vi "Untitled 1.vi"() -> ()   [LabVIEW 2021]
uses:
  <vilib>/numeric/Random Number (Range) U64.vi
  <vilib>/numeric/sub_Random U32.vi
panel:
  out "Tank":dbl(slide) scale=0.0..10.0
  in  "stop 2":bool
  out "Boolean":bool
  out "Knob":dbl(knob) scale=0.0..10.0
  out "Numeric":i32
  in  "stop":bool
  out "number":u64
  out "x+1":i32
  # "For loop"
  # "While loop"
  # "Example: Flat and stacked structures"
  # "Exercise 6"
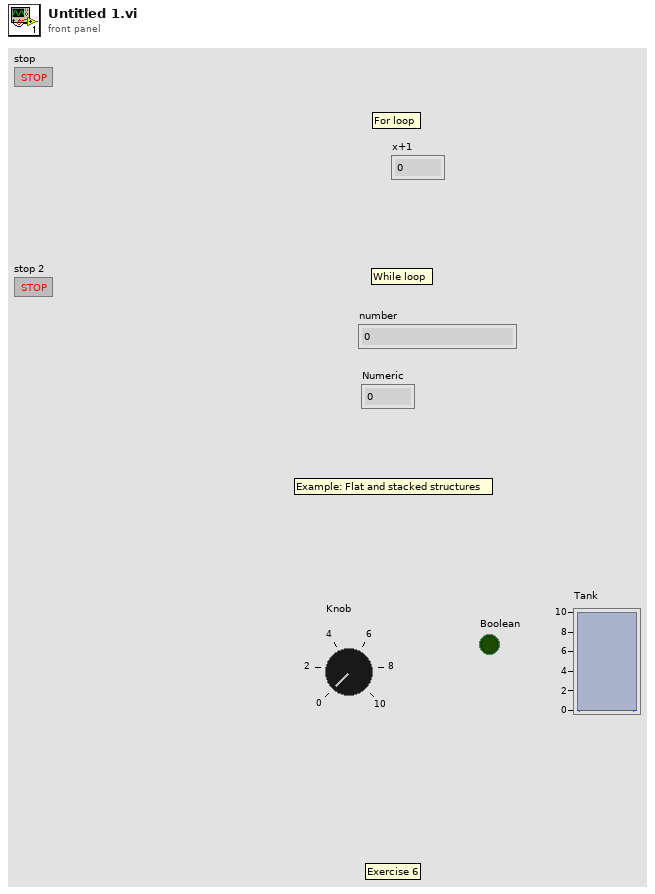
[diagram p1: front panel]
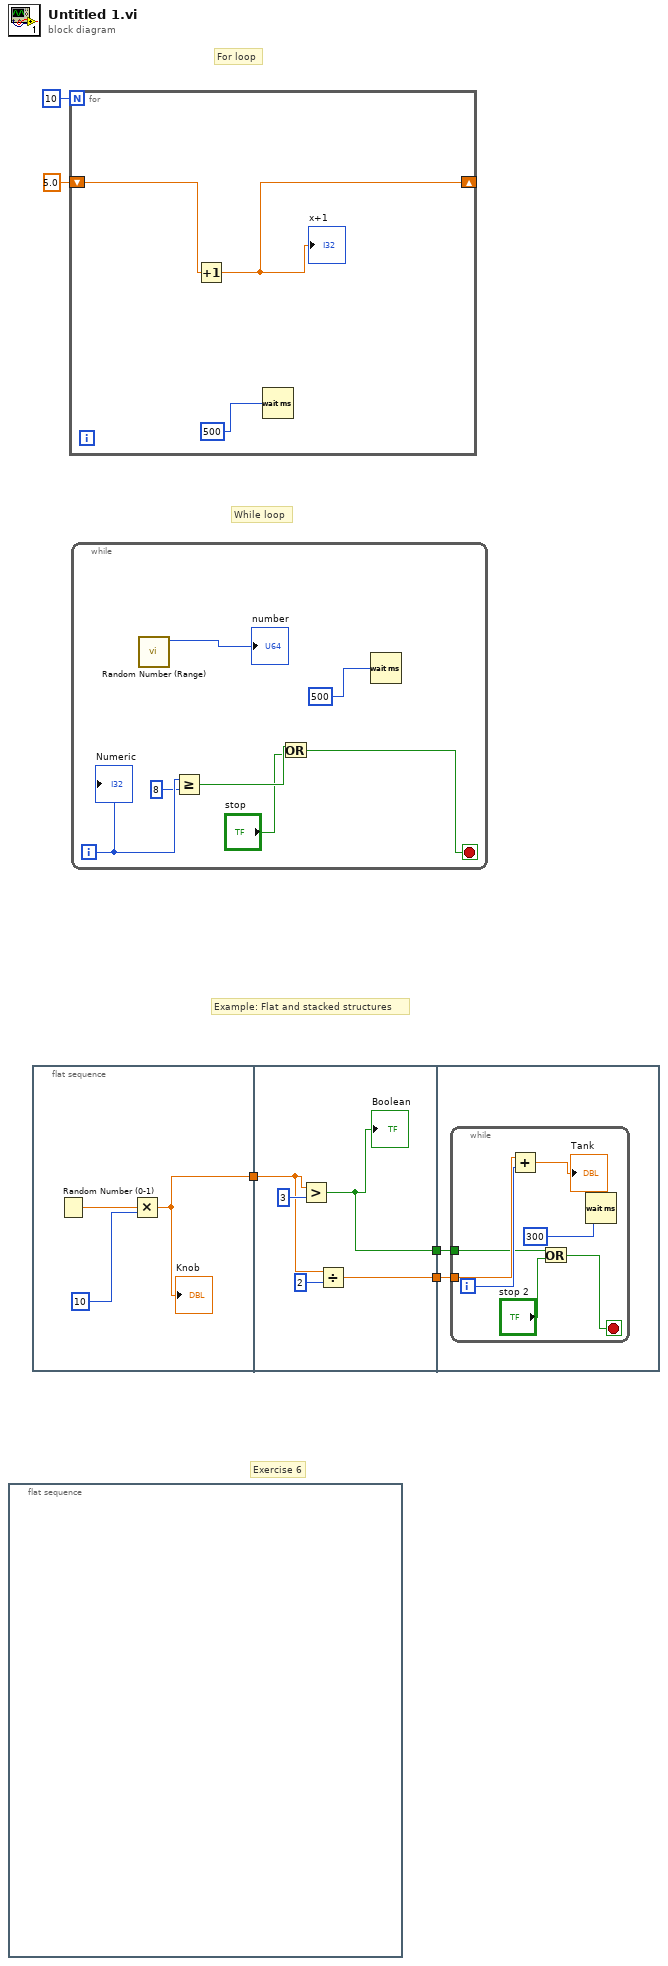
[diagram p0: block diagram]
diagram:
  # "Exercise 6"
  # "Example: Flat and stacked structures"
  # "While loop"
  # "For loop"
  n1 = flat-sequence {
    frame #0 {
    }
  }
  n2 = flat-sequence {
    tunnel: [w7] -> w3
    tunnel: w3 -> [w12]
    tunnel: [w10] -> w2
    tunnel: [w9] -> w1
    tunnel: w2 -> [w15]
    tunnel: w1 -> [w14]
    frame #0 {
      n3 = Random Number (0-1)() -> (number: 0 to 1=w6:dbl)
      n4 = Multiply(x=w6, y=u64 10) -> (x*y=w7:dbl)
      "Knob" <- w7
    }
    frame #1 {
      n5 = Greater?(x=w12, y=u64 3) -> (0:w9:bool)
      "Boolean" <- w9
      n6 = Divide(x=w12, y=u64 2) -> (x/y=w10:dbl)
    }
    frame #2 {
      n7 = while {
        tunnel: w15 -> [w21]
        tunnel: w14 -> [w20]
        i -> [w22]
        stop <- w18 stop-if-true
        n8 = Add(x=w21, y=w22) -> (x+y=→"Tank":dbl)
        n9 = Or(x=w20, y="stop 2") -> (x .or. y?=w18:bool)
        n10 = Wait (ms)(milliseconds to wait=u32 300) -> ()  [unwired: 1 out]
      }
    }
  }
  n11 = for {
    N: 10 -> [_]
    shift-right: [w23] -> _
    shift-left: 5.0 -> [w24]
    n12 = Increment(x=w24) -> (x+1=w23:dbl)
    "x+1" <- w23
    n13 = Wait (ms)(milliseconds to wait=u32 500) -> ()  [unwired: 1 out]
  }
  n14 = while {
    i -> [w31]
    stop <- w27 stop-if-true
    n15 = call-poly <vilib>:"Random Number (Range).vi"() -> ("number"=→"number":u64)  [unwired: 11 in]
    n16 = Greater Or Equal?(x=w31, y=8) -> (x >= y?=w29:bool)
    n17 = Or(x=w29, y="stop") -> (x .or. y?=w27:bool)
    n18 = Wait (ms)(milliseconds to wait=u32 500) -> ()  [unwired: 1 out]
    "Numeric" <- w31
  }
